vi "plot read autoscale.vi"(8 "error in (no error)":errorcluster, 11 "Refs":T2) -> (0 "error out":errorcluster, 3 "scale fits":T1)   [LabVIEW 2021, in "RocketPlot.lvlib"]
uses:
  RocketPlot.lvlib
  TypeDefs/Plot UI references.ctl
  Classes/RocketPlotHandle/RocketPlotHandle.lvclass
  <userlib>/bjustice/TipStripOOPanel/Classes/TipPanelHandle/TipPanelHandle.lvclass
  TypeDefs/Plot top row.ctl
  TypeDefs/plotBG inputs.ctl
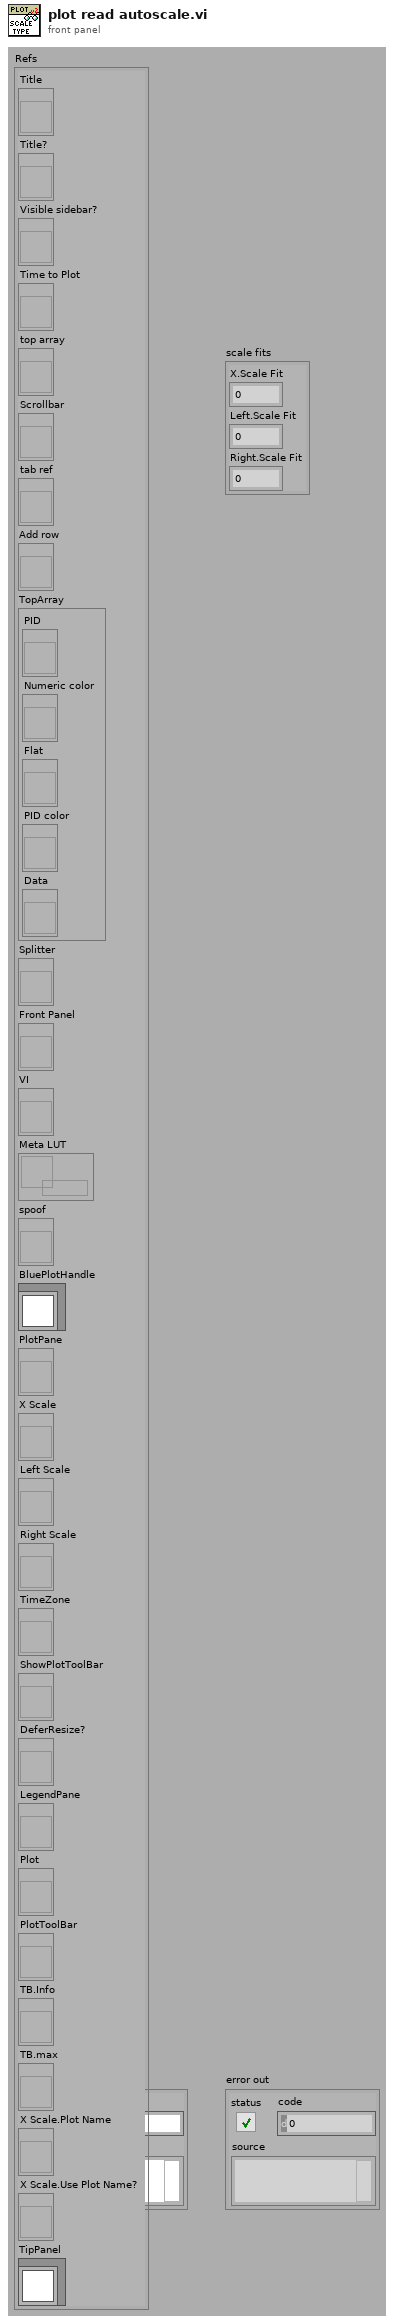
[diagram p1: front panel]
types:
  T1 = typedef "RocketPlot.lvlib/plotBG inputs.ctl" = cluster{"X.Scale Fit":u8, "Left.Scale Fit":u8, "Right.Scale Fit":u8}
  T2 = typedef "RocketPlot.lvlib/Plot UI references.ctl" = cluster{"Title":refnum<vi>, "Title?":refnum<vi>, "Visible sidebar?":refnum<vi>, "Time to Plot":refnum<vi>, "top array":refnum<vi>, "Scrollbar":refnum<vi>, "tab ref":refnum<vi>, "Add row":refnum<vi>, "TopArray":cluster{"PID":refnum<vi>, "Numeric color":refnum<vi>, "Flat":refnum<vi>, "PID color":refnum<vi>, "Data":refnum<vi>}, "Splitter":refnum<vi>, "Front Panel":refnum<vi>, "VI":refnum<vi>, "Meta LUT":refnum<data-value>, "spoof":refnum<vi>, "BluePlotHandle":refnum<class "RocketPlotHandle.lvclass">, "PlotPane":refnum<vi>, "X Scale":refnum<vi>, "Left Scale":refnum<vi>, "Right Scale":refnum<vi>, "TimeZone":refnum<vi>, "ShowPlotToolBar":refnum<vi>, "DeferResize?":refnum<vi>, "LegendPane":refnum<vi>, "Plot":refnum<vi>, "PlotToolBar":refnum<vi>, "TB.Info":refnum<vi>, "TB.max":refnum<vi>, "X Scale.Plot Name":refnum<vi>, "X Scale.Use Plot Name?":refnum<vi>, "TipPanel":refnum<class "TipPanelHandle.lvclass">}
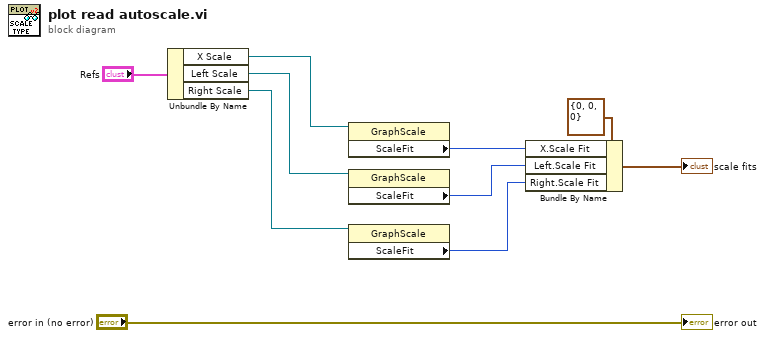
[diagram p0: block diagram]
diagram:
  n1 = Unbundle By Name("Refs") -> ("X Scale"=w9:refnum<vi>, "Left Scale"=w8:refnum<vi>, "Right Scale"=w7:refnum<vi>)
  n2 = property class="GraphScale"(reference=w9) -> ("ScaleFit"=w5:u8)  [unwired: 1 in, 2 out]
  n3 = property class="GraphScale"(reference=w8) -> ("ScaleFit"=w4:u8)  [unwired: 1 in, 2 out]
  n4 = property class="GraphScale"(reference=w7) -> ("ScaleFit"=w3:u8)  [unwired: 1 in, 2 out]
  n5 = Bundle By Name(cluster=T1 {"X.Scale Fit"=0, "Left.Scale Fit"=0, "Right.Scale Fit"=0} ("scale locked?"), "X.Scale Fit"=w5, "Left.Scale Fit"=w4, "Right.Scale Fit"=w3) -> (→"scale fits":T1)
  "error out" <- "error in (no error)"
